vi "state.vi"(11 "State":i16) -> (3 "狀態":string)   [LabVIEW 2019]
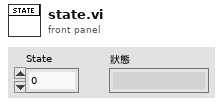
[diagram p1: front panel]
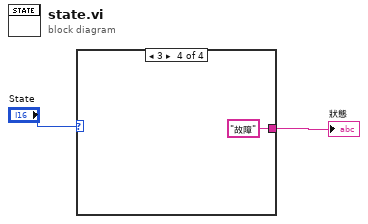
[diagram p0: block diagram]
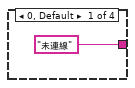
[diagram p2: hidden frame]
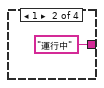
[diagram p3: hidden frame]
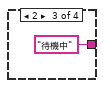
[diagram p4: hidden frame]
diagram:
  n1 = case shown="3" "State" {
    tunnel: ["未連線" "運行中" "待機中" "故障"] -> w2
    frame 0, Default {
    }
    frame 1 {
    }
    frame 2 {
    }
    frame 3 {
    }
  }
  "狀態" <- w2
